vi "niDTS BT INSTR TX UTIL Measurement Interval.vi"(7 "Measurement Length mode":enum16{"AUTO", "MANUAL"}(ring)) -> (8 "INTerval":T1)   [LabVIEW 2015, in "niDTS BT.lvlib" / "niDTS BT INSTR TX.lvclass"]
uses:
  niDTS BT INSTR TX.lvclass
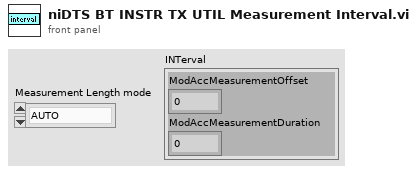
[diagram p1: front panel]
types:
  T1 = cluster{"ModAccMeasurementOffset":i32, "ModAccMeasurementDuration":i32}
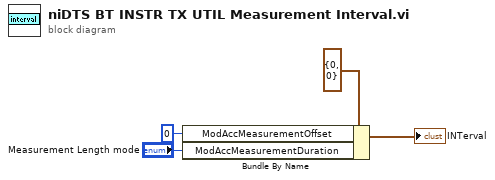
[diagram p0: block diagram]
diagram:
  n1 = Bundle By Name(cluster=T1 {"ModAccMeasurementOffset"=0, "ModAccMeasurementDuration"=0} ("INTerval"), "ModAccMeasurementOffset"=0, "ModAccMeasurementDuration"="Measurement Length mode") -> (→"INTerval":T1)
